vi "GetDisplayProperties.vi"(8 "No Error":errorcluster, 11 "Display ID":T2) -> (0 "Error Out":errorcluster, 3 "PropertiesID":T1)   [LabVIEW 2026, in "SDL3.lvlib" / "Video.lvlib"]
doc: "<B>Summary</B>\nGet the properties associated with a display.\n\n<B>Remarks</B>\nThe following read-only properties are provided by SDL:\n\n- <B>SDL_PROP_DISPLAY_HDR_ENABLED_BOOLEAN</B>: true if the display has HDR headroom above the SDR white point. This is for informational and diagnostic purposes only, as not all platforms provide this information at the display level.\n\nOn KMS/DRM:\n- <B>SDL_PROP_DISPLAY_KMSDRM_PANEL_ORIENTATION_NUMBER</B>: the \"panel orientation\" property for the display in degrees of clockwise rotation. Note that this is provided only as a hint, and the application is responsible for any coordinate transformations needed to conform to the requested display orientation."
uses:
  Video.lvlib
  DisplayID--integer.ctl
  Properties/PropertiesID--integer.ctl
  <vilib>/Utility/error.llb/Error Cluster From Error Code.vi
  Error/Error.lvlib
  Lib/SDL3.dll
  Properties/Properties.lvlib
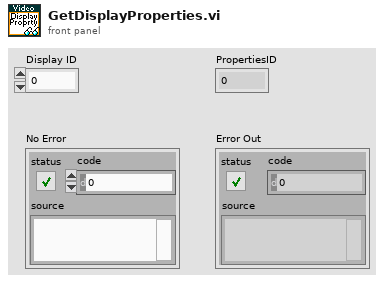
[diagram p1: front panel]
types:
  T1 = typedef "SDL3.lvlib/Properties.lvlib/PropertiesID--integer.ctl" = u32
  T2 = typedef "SDL3.lvlib/Video.lvlib/DisplayID--integer.ctl" = u32
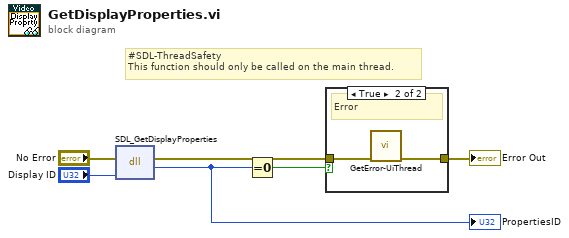
[diagram p0: block diagram]
diagram:
  # "#SDL-ThreadSafety\nThis function should only be called on the main thread."
  n1 = dll-call lib="C:/Users/saukko/Dev/LV-SDL3/Sources/SDL3/Lib/SDL3.*" fn="SDL_GetDisplayProperties"(error in="No Error", "displayID"="Display ID") -> (error out=w3:errorcluster, "return type"=w1:u32)  [unwired: 3 in, 1 out]
  "PropertiesID" <- w1
  n2 = Equal To 0?(x=w1) -> (x = 0?=w2:bool)
  n3 = case shown="True" w2 {
    tunnel: w3 -> [w7 w9]
    tunnel: [w7 w8] -> w5
    frame False {
      # "Ok"
    }
    frame True {
      # "Error"
      n4 = call "GetError-UiThread.vi"("No Error"=w9) -> ("error out"=w8:errorcluster)  [unwired: 10 in]
    }
  }
  "Error Out" <- w5
